vi "Read Multi Eval Meas Trace EVM Vs Subcarrier Results.vi"(8 "error in (no error)":errorcluster, 10 "Instance (1)":T1=1, 11 "VISA resource name":refnum<visa-resource-name>) -> (0 "error out":errorcluster, 1 "EVM Vs Subcarrier Results":dbl[](array[numeric]) format="%^.3e", 2 "Reliability":i32, 3 "VISA resource name out":refnum<visa-resource-name>)   [LabVIEW 2020, in "Rohde&Schwarz CMXP NR FR2 Measurement.lvlib"]
doc: "Starts a new single shot measurement and returns the multi eval measurement EVM vs subcarrier trace.\n\nAttribute:\nRSCMXPNRFR2M_ATTR_READ_MULTI_EVAL_MEASUREMENT_TRACE_EVM_VS_SUBCARRIER_RESULTS\n\nRemote-control command:\nREAD:NRMMw:MEAS<i>:MEValuation:TRACe:EVMC?"
uses:
  <instrlib>/Rohde&Schwarz CMXP NR FR2 Measurement/Rohde&Schwarz CMXP NR FR2 Measurement.lvlib
  <instrlib>/Rohde&Schwarz CMXP NR FR2 Measurement/Private/_Instance.ctl
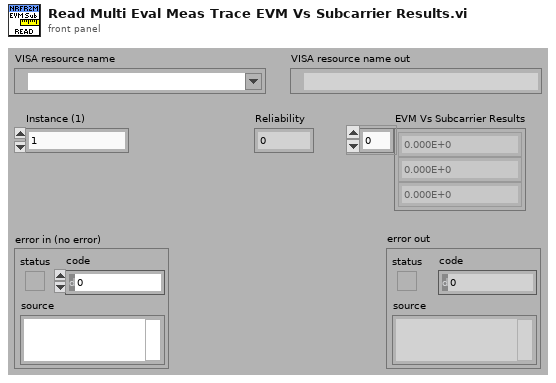
[diagram p1: front panel]
types:
  T1 = typedef "Rohde&Schwarz CMXP NR FR2 Measurement.lvlib/_Instance.ctl" = i32
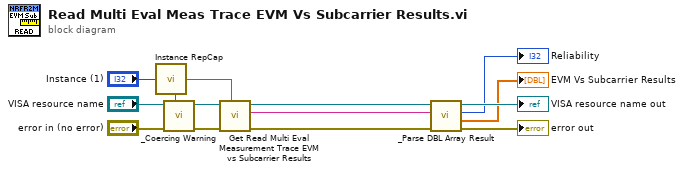
[diagram p0: block diagram]
diagram:
  n1 = call <instrlib>:"Instance RepCap.vi"("Instance In"="Instance (1)") -> ("In Range?"=w4:bool, "RepCap Identifier Out"=w7:string)  [unwired: 1 in]
  n2 = call <instrlib>:"_Coercing Warning.vi"("In Range?"=w4, "error in (no error)"="error in (no error)", "VISA resource name"="VISA resource name") -> ("error out"=w2:errorcluster, "VISA resource name out"=w3:refnum<visa-resource-name>)  [unwired: 7 in]
  n3 = call "Get Read Multi Eval Measurement Trace EVM vs Subcarrier Results"("Repeated Capabilities"=w7, "error in (no error)"=w2, "instrument handle"=w3) -> ("error out"=w12:errorcluster, "Read Multi Eval Measurement Trace EVM vs Subcarrier Results"=w13:string, "instrument handle out"=w14:refnum<visa-resource-name>)  [unwired: 6 in]
  n4 = call <instrlib>:"_Parse DBL Array Result.vi"("error in (no error)"=w12, "Input String"=w13, "VISA resource name"=w14) -> ("error out"=→"error out":errorcluster, "Results"=→"EVM Vs Subcarrier Results":dbl[], "Reliability"=→"Reliability":i32, "VISA resource name out"=→"VISA resource name out":refnum<visa-resource-name>)  [unwired: 5 in]
